vi "Instantiate Class.vi"(8 "error in (no error)":errorcluster, 11 "String":string) -> (0 "error out":errorcluster, 3 "LabVIEW Object out":refnum<class>)   [LabVIEW 2018, in "Configuration File.lvlib" / "Configuration File.lvclass"]
doc: "This VI instantiates an object of a class based on the input string. For this VI to load the class correctly, the library owning the class must be loaded in memory for LabVIEW to find it. It will send an error detailing whwere the class was not able to instantiate."
uses:
  Configuration File.lvclass
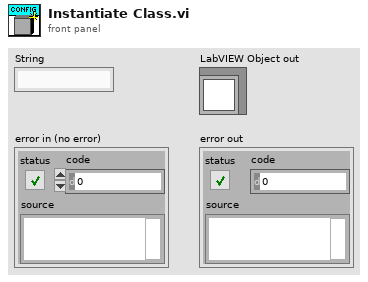
[diagram p1: front panel]
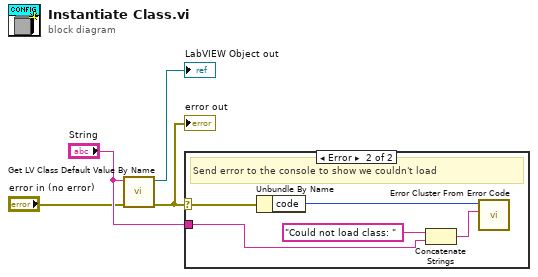
[diagram p0: block diagram]
diagram:
  n1 = call <vilib>:"Get LV Class Default Value By Name.vi"("error in (no error)"="error in (no error)", "class name"="String") -> ("error out"=w3:errorcluster, "object"=→"LabVIEW Object out":refnum<class>)  [unwired: 8 in]
  "error out" <- w3
  n2 = case shown="Error" w3 {
    selector: w3 -> [_ w6]
    tunnel: "String" -> [_ w5]
    frame No Error {
    }
    frame Error {
      # "Send error to the console to show we couldn't load"
      n3 = Unbundle By Name(w6) -> ("code"=w7:i32)
      n4 = Concatenate Strings("Could not load class: " ("error message (\"\")"), w5) -> (w8:string)
      n5 = call <vilib>:"Error Cluster From Error Code.vi"("error message (\"\")"=w8, "error code (0)"=w7) -> ()  [unwired: 7 in, 1 out]
    }
  }
